vi "Test Cameras.vi"(8 "error in":errorcluster, 11 "Session In":T1) -> (0 "error out":errorcluster, 3 "Valid Camera":bool)   [LabVIEW 2016]
doc: "Tests a camera session and returns the validty (True:Valid)"
uses:
  <vilib>/userdefined/High Color/IMAQdx.ctl
  <vilib>/vision/driver/NI_Vision_Acquisition_Software.lvlib
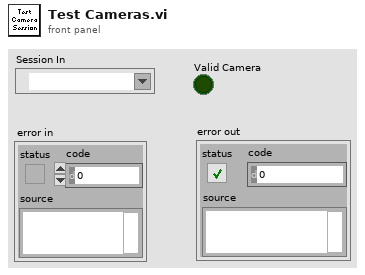
[diagram p1: front panel]
types:
  T1 = typedef "IMAQdx.ctl" = refnum<k21>
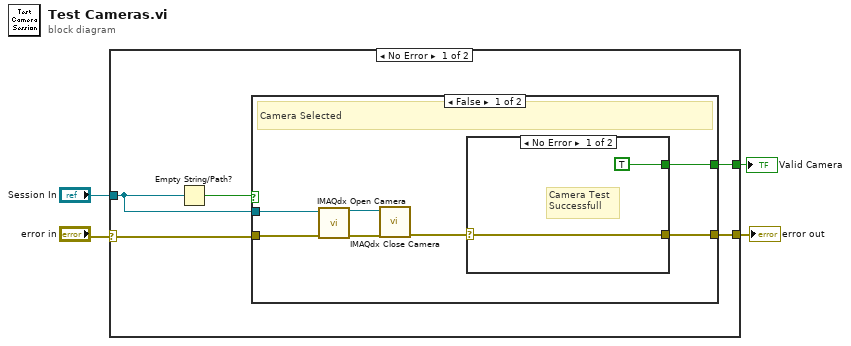
[diagram p0: block diagram]
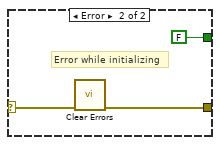
[diagram p2: hidden frame]
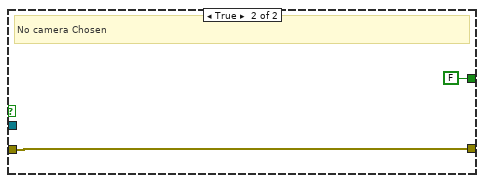
[diagram p3: hidden frame]
diagram:
  n1 = case shown="No Error" "error in" {
    selector: "error in" -> [w7 w24]
    tunnel: [w8 _] -> w4
    tunnel: "Session In" -> [w6 _]
    tunnel: [w5 w24] -> w1
    frame No Error {
      n2 = Empty String/Path?(string/path=w6) -> (empty?=w9:bool)
      n3 = case shown="False" w9 {
        tunnel: w6 -> [w16 _]
        tunnel: [w12 FALSE] -> w8
        tunnel: w7 -> [w11 w23]
        tunnel: [w10 w23] -> w5
        frame False {
          # "Camera Selected"
          n4 = call <vilib>:"IMAQdx Open Camera.vi"("error in"=w11, "Session In"=w16) -> ("error out"=w14:errorcluster, "Session Out"=w15:T1)  [unwired: 8 in]
          n5 = call <vilib>:"IMAQdx Close Camera.vi"("error in"=w14, "Session In"=w15) -> ("error out"=w13:errorcluster)  [unwired: 9 in]
          n6 = case shown="No Error" w13 {
            selector: w13 -> [w17 w20]
            tunnel: [TRUE FALSE] -> w12
            tunnel: [w17 w19] -> w10
            frame No Error {
              # "Camera Test \nSuccessfull"
            }
            frame Error {
              # "Error while initializing"
              n7 = call <vilib>:"Clear Errors.vi"("error in (no error)"=w20) -> ("error out"=w19:errorcluster)  [unwired: 5 in, 1 out]
            }
          }
        }
        frame True {
          # "No camera Chosen"
        }
      }
    }
    frame Error {
      # "Error detected"
    }
  }
  "Valid Camera" <- w4
  "error out" <- w1
